vi "Begin.vi"(8 "error in (no error)":errorcluster, 10 "Settings":variant, 11 "Simulated Drive in":refnum<class "Simulated Drive.lvclass">) -> (0 "error out":errorcluster, 3 "Simulated Drive out":refnum<class "Simulated Drive.lvclass">)   [LabVIEW 2019, in "DriveOld.lvlib" / "Simulated Drive.lvclass"]
doc: "This VI holds the begin code"
uses:
  Simulated Drive.lvclass
  Drive.lvclass
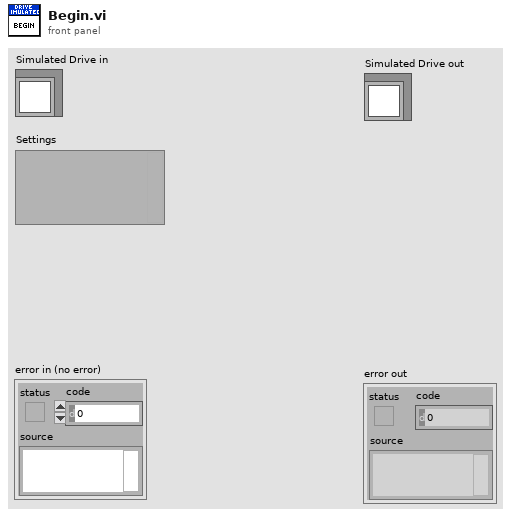
[diagram p1: front panel]
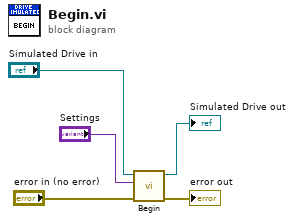
[diagram p0: block diagram]
diagram:
  n1 = call-parent "Begin.vi"("error in (no error)"="error in (no error)", "Settings"="Settings", "Drive in"="Simulated Drive in") -> ("error out"=→"error out":errorcluster, "Drive out"=→"Simulated Drive out":refnum<class "Simulated Drive.lvclass">)  [unwired: 7 in]
